vi "zadanie_2.vi"() -> ()   [LabVIEW 2020]
panel:
  in  "stop":bool
  out "2":bool
  out "1":bool
  in  "2":bool
  in  "1":bool
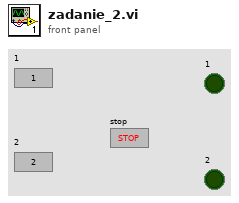
[diagram p1: front panel]
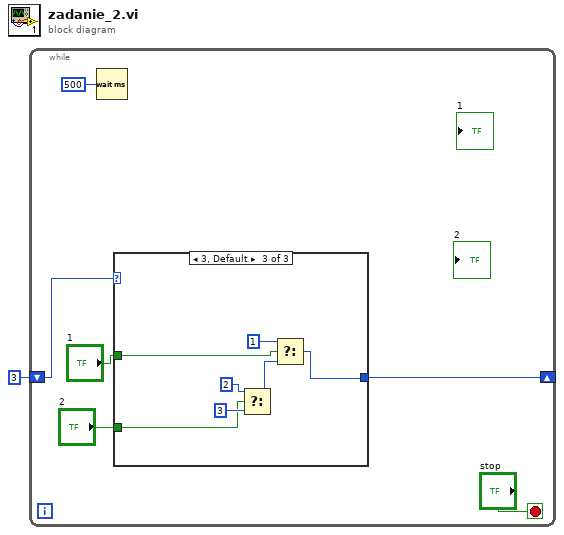
[diagram p0: block diagram]
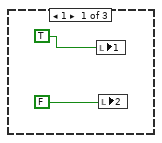
[diagram p2: hidden frame]
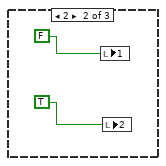
[diagram p3: hidden frame]
diagram:
  n1 = while {
    shift-right: [w5] -> _
    shift-left: 3 ("f") -> [w4]
    stop <- "stop" stop-if-true
    n2 = Wait (ms)(milliseconds to wait=u32 500) -> ()  [unwired: 1 out]
    n3 = case shown="3, Default" w4 {
      tunnel: [_ _ w14] -> w5
      tunnel: "2" -> [_ _ w13]
      tunnel: "1" -> [_ _ w12]
      frame 1 {
        n4 = local write "1"(TRUE) -> ()
        n5 = local write "2"(FALSE) -> ()
      }
      frame 2 {
        n6 = local write "1"(FALSE) -> ()
        n7 = local write "2"(TRUE) -> ()
      }
      frame 3, Default {
        n8 = Select(t=2, s=w13, f=3) -> (s? t:f=w16:i32)
        n9 = Select(t=1, s=w12, f=w16) -> (s? t:f=w14:i32)
      }
    }
  }
